vi "Read id.vi"(8 "error in (no error)":errorcluster, 11 "DSFTransfer in":refnum<class "DSFTransfer.lvclass">) -> (0 "error out":errorcluster, 2 "id":string, 3 "DSFTransfer out":refnum<class "DSFTransfer.lvclass">)   [LabVIEW 2017, in "DSFTransfer.lvclass"]
uses:
  DSFTransfer.lvclass
  DSFTransfer.lvclass/DSFTransfer.ctl
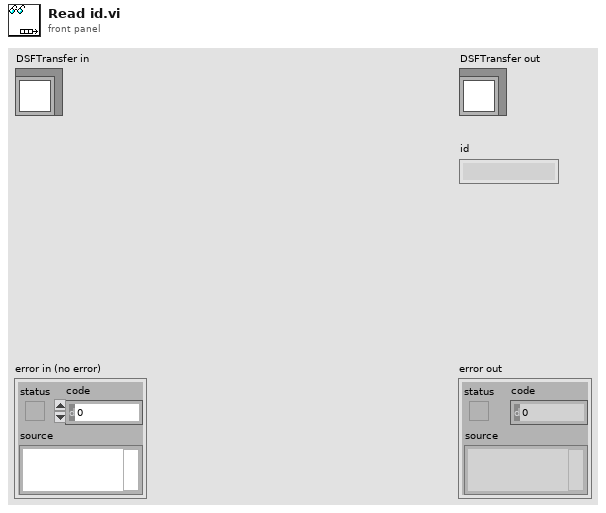
[diagram p1: front panel]
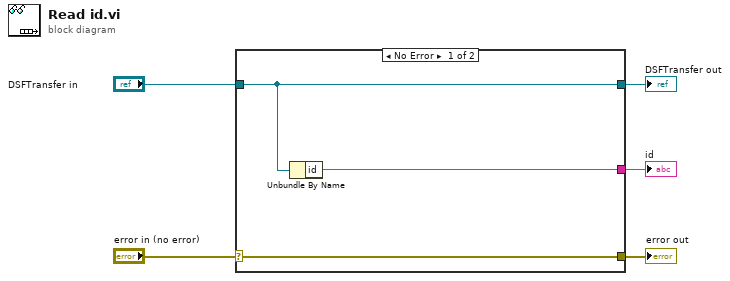
[diagram p0: block diagram]
diagram:
  n1 = case shown="No Error" "error in (no error)" {
    selector: "error in (no error)" -> [w8 w9]
    tunnel: [w8 w9] -> w4
    tunnel: [w7 w10] -> w2
    tunnel: "DSFTransfer in" -> [w7 w10]
    tunnel: [w6 _] -> w1
    frame No Error {
      n2 = Unbundle By Name(w7) -> ("id"=w6:string)
    }
    frame Error {
    }
  }
  "error out" <- w4
  "DSFTransfer out" <- w2
  "id" <- w1
